vi "score sorter.vi"(3 "Array 2":cluster{"Numeric":dbl, "Numeric 2":i32}[](array[cluster])) -> (1 "Array":cluster{"Numeric":dbl, "Numeric 2":dbl}[](array[cluster]))   [LabVIEW 2014]
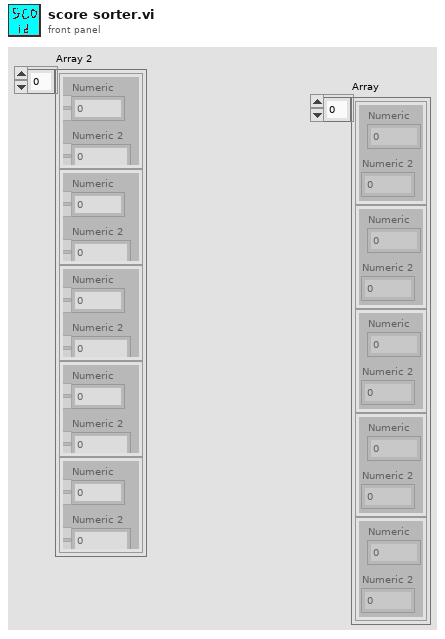
[diagram p1: front panel]
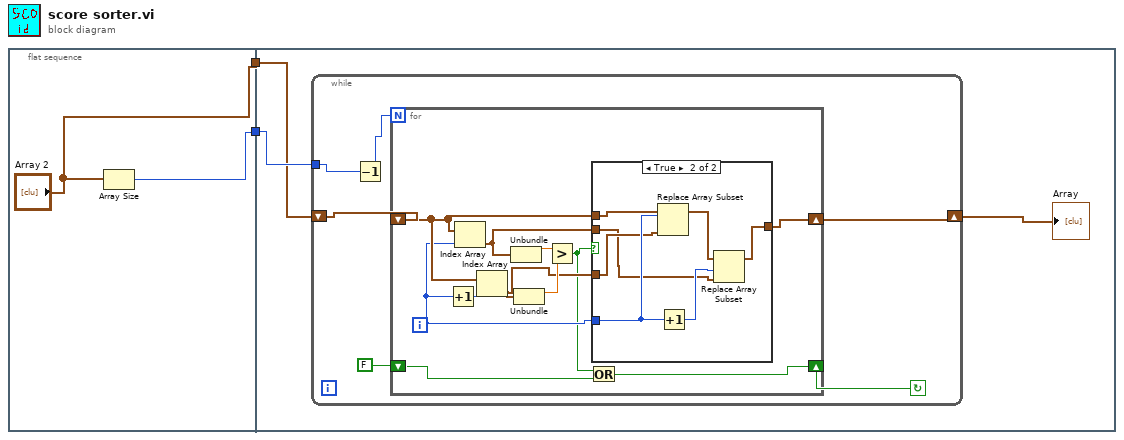
[diagram p0: block diagram]
diagram:
  n1 = flat-sequence {
    tunnel: [w4] -> w2
    tunnel: ["Array 2"] -> w1
    tunnel: w2 -> [w7]
    tunnel: w1 -> [w6]
    frame #0 {
      n2 = Array Size(array="Array 2") -> (size(s)=w4:i32)
    }
    frame #1 {
      n3 = while {
        shift-right: [w8] -> w5
        shift-left: w6 -> [w13]
        tunnel: w7 -> [w10]
        stop <- w11 continue-if-true
        n4 = Decrement(x=w10) -> (x-1=w9:i32)
        n5 = for {
          N: w9 -> [_]
          shift-right: [w19] -> w8
          shift-left: w13 -> [w21]
          shift-right: [w23] -> w11
          shift-left: FALSE -> [w22]
          i -> [w20]
          n6 = Increment(x=w20) -> (x+1=w24:i32)
          n7 = Index Array(array=w21, index=w20) -> (element=w18:cluster{"Numeric":dbl, "Numeric 2":i32})
          n8 = Index Array(array=w21, index=w24) -> (element=w15:cluster{"Numeric":dbl, "Numeric 2":i32})
          n9 = Unbundle(w18) -> ("Numeric"=w17:dbl)  [unwired: 1 out]
          n10 = Unbundle(w15) -> ("Numeric"=w16:dbl)  [unwired: 1 out]
          n11 = Greater?(x=w17, y=w16) -> (0:w14:bool)
          n12 = Or(x=w14, y=w22) -> (x .or. y?=w23:bool)
          n13 = case shown="True" w14 {
            tunnel: w21 -> [w25 w32]
            tunnel: w20 -> [_ w31]
            tunnel: w18 -> [_ w26]
            tunnel: [w25 w28] -> w19
            tunnel: w15 -> [_ w27]
            frame False {
            }
            frame True {
              n14 = Replace Array Subset(array=w32, new element=w27, index=w31) -> (w30:cluster{"Numeric":dbl, "Numeric 2":i32}[])
              n15 = Increment(x=w31) -> (x+1=w29:i32)
              n16 = Replace Array Subset(array=w30, new element=w26, index=w29) -> (w28:cluster{"Numeric":dbl, "Numeric 2":i32}[])
            }
          }
        }
      }
      "Array" <- w5
    }
  }
